vi "serial_log.vi"(7 "filename prefix":string, 8 "Read":string, 9 "ReadByte":i32, 10 "Send":string, 11 "SendByte":i32) -> ()   [LabVIEW 2019]
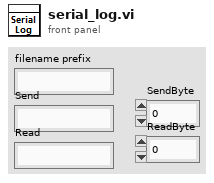
[diagram p1: front panel]
types:
  T1 = enum16{"open", "replace", "create", "open or create", "replace or create", "replace or create with confirmation"}
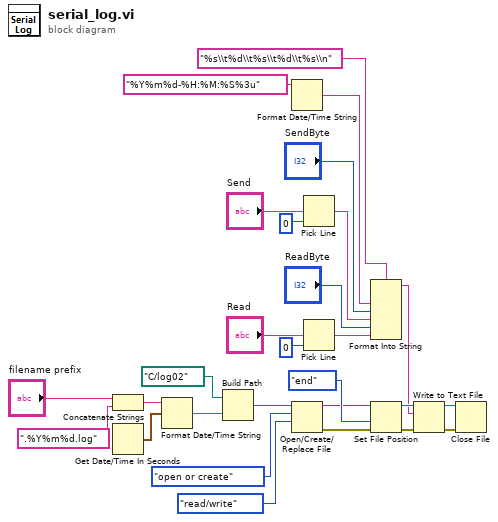
[diagram p0: block diagram]
diagram:
  n1 = Concatenate Strings("filename prefix", ".%Y%m%d.log" ("time format string (%c)")) -> (w14:string)
  n2 = Get Date/Time In Seconds() -> (seconds since 1Jan1904=w17:timestamp)
  n3 = Format Date/Time String(time format string (%c)=w14, seconds (now)=w17) -> (date/time string=w16:string)  [unwired: 1 in]
  n4 = Build Path(base path=path "C:/log02" ("file path (use dialog)"), name or relative path=w16) -> (appended path=w19:path)
  n5 = Format Date/Time String(time format string (%c)="%Y%m%d-%H:%M:%S%3u") -> (date/time string=w7:string)  [unwired: 2 in]
  n6 = Open/Create/Replace File(file path (use dialog)=w19, operation (0:open)=T1."open or create", access (0:read/write)=enum16{"read/write", "read-only", "write-only"}."read/write") -> (refnum out=w26:refnum<file>, error out=w24:errorcluster)  [unwired: 3 in, 1 out]
  n7 = Pick Line(multi-line string="Send", line index=0) -> (output string=w6:string)  [unwired: 1 in]
  n8 = Pick Line(multi-line string="Read", line index=0) -> (output string=w5:string)  [unwired: 1 in]
  n9 = Format Into String(format string="%s\\t%d\\t%s\\t%d\\t%s\\n", w7, "SendByte", w6, "ReadByte", w5) -> (resulting string=w1:string)  [unwired: 2 in, 1 out]
  n10 = Set File Position(refnum=w26, from (0:start)=enum16{"start", "end", "current"}."end", error in=w24) -> (refnum out=w25:refnum<file>, error out=w23:errorcluster)  [unwired: 1 in]
  n11 = Write to Text File(file (use dialog)=w25, text=w1, error in=w23) -> (refnum out=w22:refnum<file>, error out=w21:errorcluster)  [unwired: 1 in, 1 out]
  n12 = Close File(refnum=w22, error in=w21) -> ()  [unwired: 2 out]
